vi "CV.vi"(2 "Run uninterrupted?":bool, 3 "Device Category IN:":string(combo)="ATLAS18SS" caption="Device Category:", 4 "Batch No.:":string, 5 "Sensor Serial No.:":string, 6 "DB Serial No.:":string) -> (0 "Done!":bool)   [LabVIEW 2019]
doc: "Performs CV measurements according to ATLAS ITk Quality Control Specifications."
uses:
  general_VIs/globals/QC_MeasurementSetup.vi
  general_VIs/globals/QC_RunInformation.vi
  InstrControl/InstrumentSetup.vi
  InstrControl/Switching/Switching.lvclass
  InstrControl/SupplyControl/SupplyControl.lvclass
  InstrControl/LCRControl/LCRControl.lvclass
  InstrControl/ArduinoControl/ArduinoControl.lvclass
  <vilib>/Analysis/NI_AALBase.lvlib
  InstrControl/InstrControl.lvclass
panel:
  out "Measurement Configuration Tab":enum32{"CV Setup", "CV Scan"}(tab)
  in  "V_depletion limit [V]":dbl=-300.0
  in  "step interval [s] IN":i32=5 caption="step interval [s]"
  in  "step [V] IN":dbl=10.0 caption="step [V]" format="%.1f"
  in  "Final volts [V] IN":dbl=-500.0 caption="Final volts [V]"
  in  "Initial volts [V] IN":dbl caption="Initial volts [V]"
  in  "Current Limit [µA]":dbl=1000.0 min=0.0001 format="%.3f"
  in  "Continue":bool
  in  "Quit":bool
  in  "Software current limit?":bool
  in  "Frequency [Hz] Setup":i32=500 caption="Frequency [Hz]" format="%#.3p"
  in  "Measurement Configurations":bool
  out "RH":dbl[](array[numeric]) caption="RH [%]" format="%#.2f"
  out "step interval [s]":u32=5
  out "step [V]":dbl=10.0 format="%.1f"
  out "Final volts [V]":dbl=-700.0 format="%.1f"
  out "Initial volts [V]":dbl format="%.1f"
  out "Frequency [Hz]":i32=1000 format="%#.3p"
  out "Temp.":dbl[](array[numeric]) caption="Temp. [°C]" format="%#.2f"
  out "Volts":dbl[](array[numeric]) caption="Volts [V]"
  out "Resistance":dbl[](array[numeric]) caption="Res [kOhm]"
  out "Capacitance":dbl[](array[numeric]) caption="Cap [pF]"
  out "Cgraph":cluster{"Initial volts":dbl, dbl, dbl[]}(graph)
  in  "Scales":T1(ring)
  in  "Cscale":enum16{"1/C^2 [1/nF^2]", "nF", "pF"}(ring)
  out "positive ramp?":bool
  out "DUT Description/Hardware Tab":enum32{"CV Setup", "CV Scan"}(tab)
  in  "Switching":string(combo)="Pickering Matrix"
  in  "LCR Meter":string(combo)="WayneKerr 6440B"
  in  "User:":string(combo)="Christoph"
  in  "CV Supply":string(combo)="Keithley 2410"
  in  "Hardware Configurations":bool
  in  "Temperature":enum16{"Read Arduino", "Enter manually"}(ring)
  in  "Manufacturer:":string(combo)="Hamamatsu"
  in  "abort":bool
  out "Device Category:":string
  out "DB Serial No.:":string
  out "Current Volts:":dbl format="%.2f"
  in  "quit (no save)":bool
  in  "Quit & Save":bool
  out "Bias On/Off:":bool
  out "STATUS 1":string
  out "Initiated:":string
  out "Sensor No.:":string
  out "No of steps":u32
  out "Current reading No.":u32
  out "Last reading at:":string
  # "Strip Sensor QC: CV"
  # "University of\nCambridge"
  # "Vertical Scale:"
  # "Measurement Configuration"
  # "CV Scan parameters:"
  # "Last 5 readings:"
  # "n-4"
  # "n-3"
  # "n-2"
  # "n-1"
  # "n"
  # "DUT Description"
  # "Hardware"
  # "DUT & Test Description:"
  # "Current status:"
  # "Rdg No:"
  # "out of"
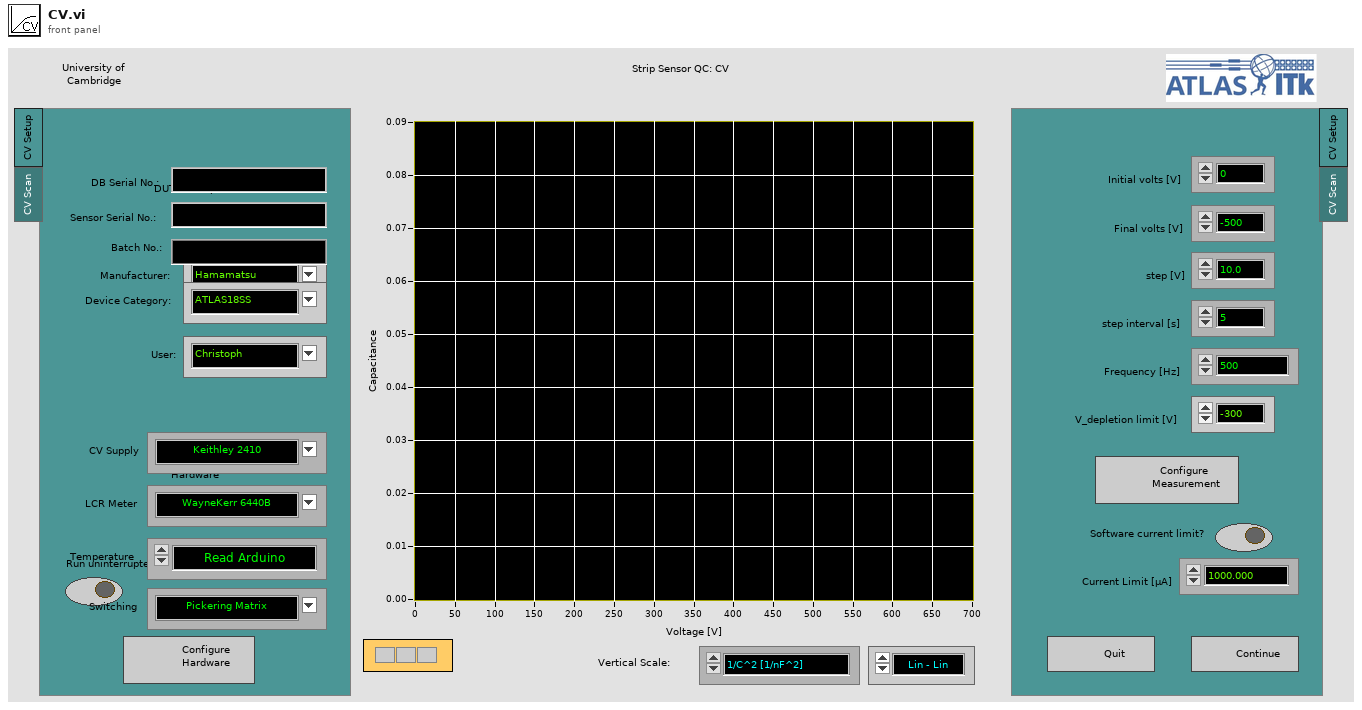
[diagram p1: front panel]
types:
  T1 = enum16{"Lin - Lin", "Log - Lin", "Lin - Log", "Log - log"}
  T2 = enum16{"Supply", "LCR", "Multimeter", "Switching"}
  T3 = enum16{"Reset", "Read Array", "Read Element", "Write Element", "Write Array", "Add Element", "Add Array"}
  T4 = enum16{"Reset", "Ground", "Striptest Bias", "Striptest SMU", "Striptest LCR", "IV", "CV", "Interstrip Cap", "Interstrip Res"}
  T5 = enum32{"IV", "CV", "Stability", "Striptest", "Cis", "Ris", "PTP"}
  T6 = cluster{"Supply":refnum<class "SupplyControl.lvclass">, "LCR":refnum<class "LCRControl.lvclass">, "Initial Voltage [V]":dbl, "Final Voltage [V]":dbl, "Step Size [V]":dbl, "Step Interval [s]":i32, "Number Of Steps":u32, "AC frequency [Hz]":i32, "RC Configuration":u16, "AC amplitude [V]":dbl, "Ramp down steps [V]":dbl, "Ramp down Interval [s]":i32, "Set Current Limit?":bool, "Current Limit [µA]":dbl, "Temperature Readout":enum16{"Read Arduino", "Enter manually"}, "Arduino":refnum<class "ArduinoControl.lvclass">, "Supply Name":string, "LCR Name":string, "V_depletion Limit [V]":dbl, "Switching":refnum<class "Switching.lvclass">, "Matrix used?":bool, "Matrix X Channels":cluster{"Bias Supply / SMU LO":i32, "Bias Supply / SMU HI":i32, "CV Box LO":i32, "CV Box HI":i32, "CV Box LO IN":i32, "CV Box HI IN":i32, "Volt meter LO":i32, "Volt meter HI":i32, "Mux1 C1":i32, "Mux1 C2":i32, "Mux2 C1":i32, "Mux2 C2":i32}}
  T7 = cluster{"Sensor Serial No.:":string, "Wafer Serial No.:":string, "Batch:":string, "Manufacturer:":string, "Device Category:":string, "Database Serial No.:":string, "Date Initiated:":string, "Time Initiated:":string, "Test":string, "Instruments used:":string, "Probeplan used:":string, "End of Run comment:":string, "User:":string}
  T8 = cluster{"Institute":string, "Manufacturers":string[], "Devices":string[], "Serialnumbers Lookup DB":string, "Data directory":string, "Backup & screenshot directory":string, "List of known users":string[], "Measurement switch not used":bool, "Measurement Switch":string, "DUT Switch":string}
  T9 = cluster{"Current Limit":sgl, "KE2410":refnum<class "KE2410.lvclass">}
  T10 = cluster{"VISA address":refnum<visa-resource-name>, "T sensor":enum16{"SHT", "DS"}, "Arduino":refnum<class "ArduinoControl.lvclass">}
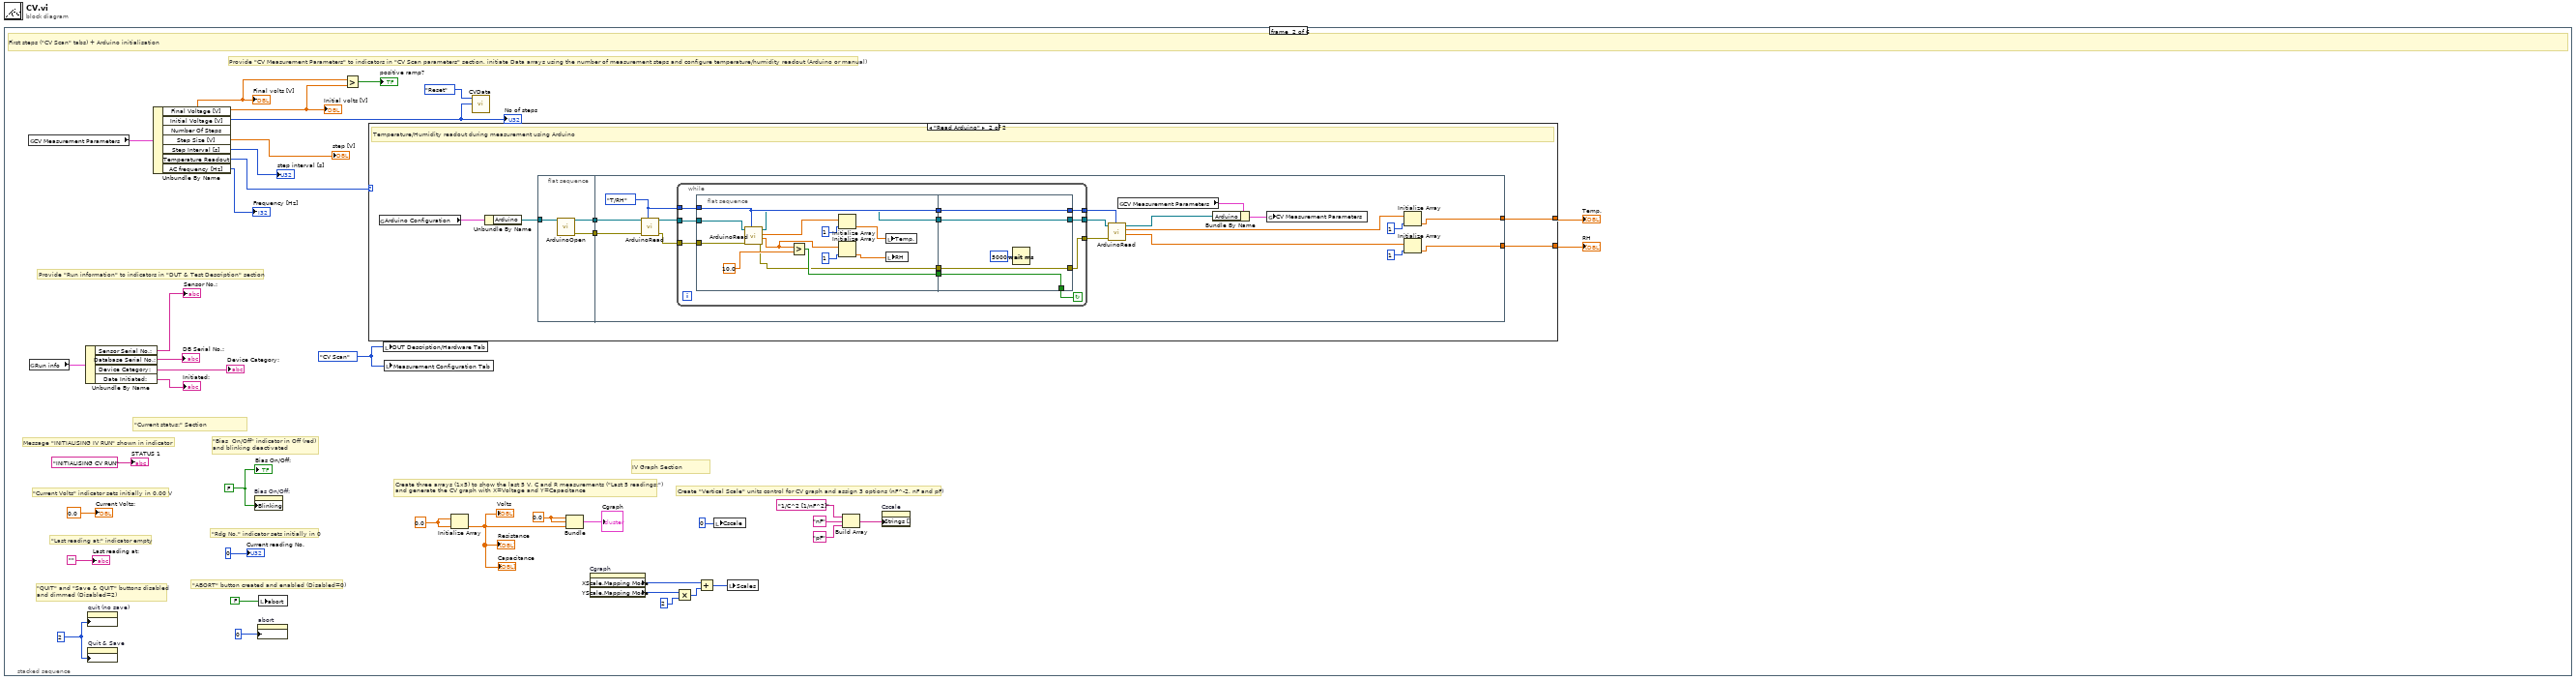
[diagram p0: block diagram]
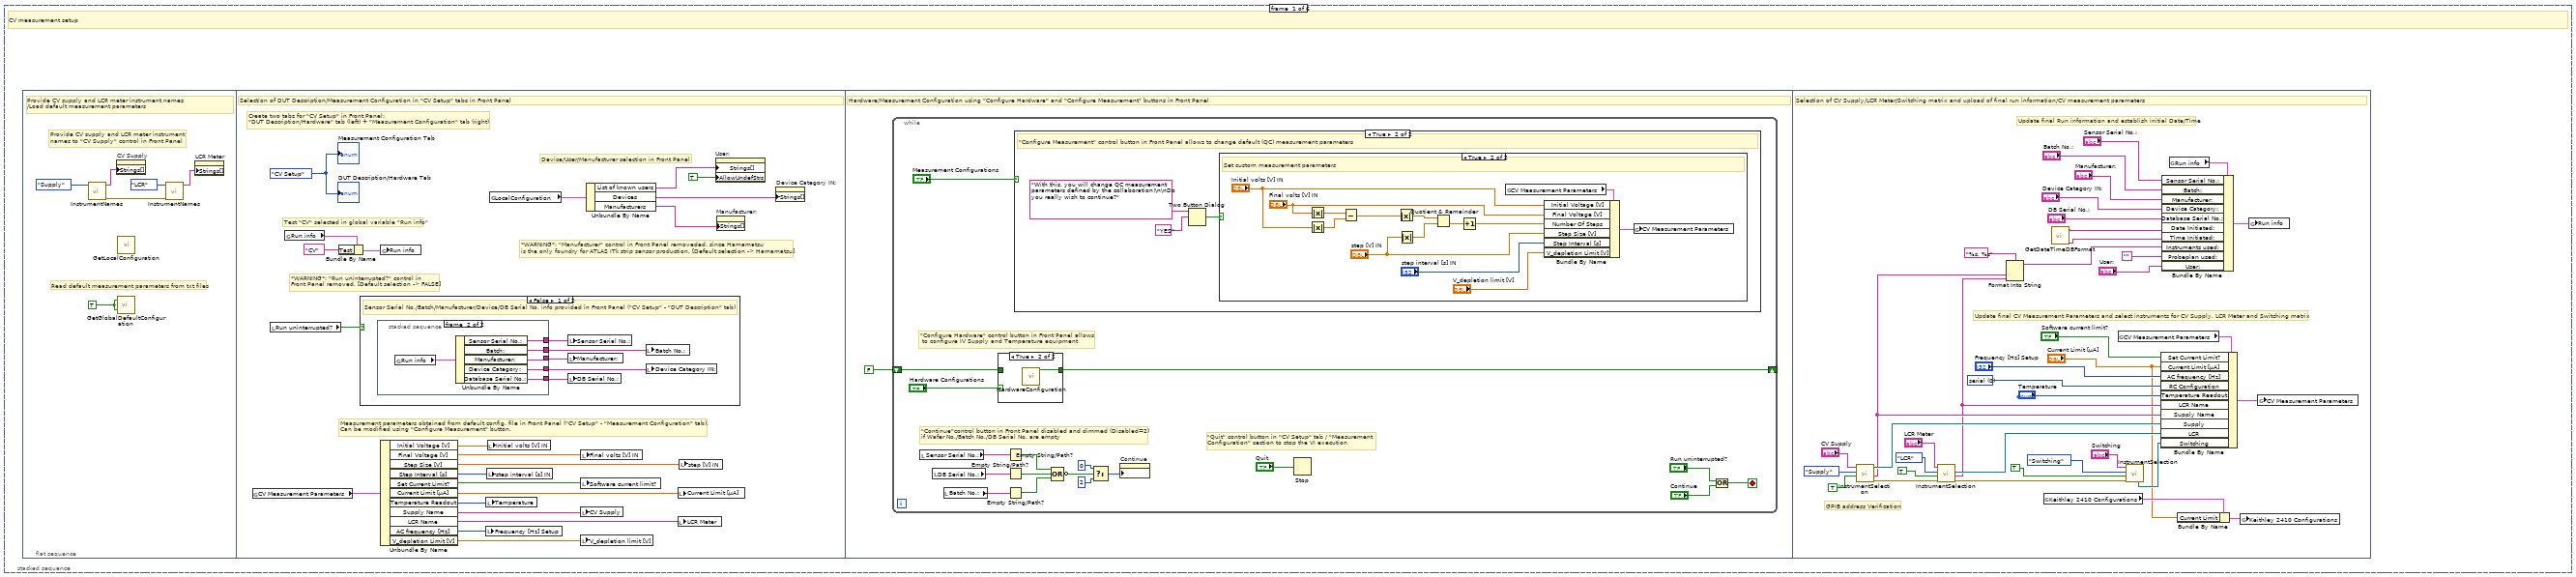
[diagram p2: hidden frame]
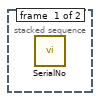
[diagram p3: hidden frame]
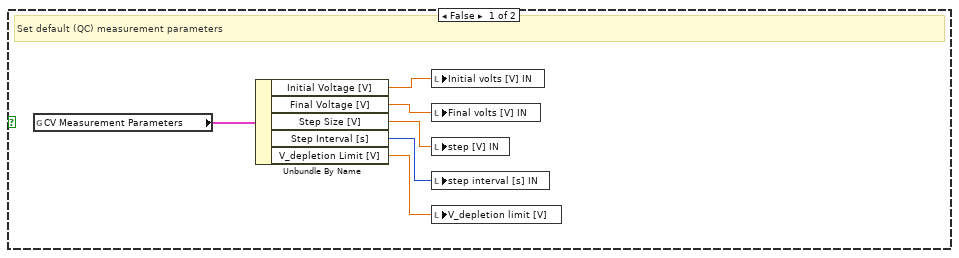
[diagram p7: hidden frame]
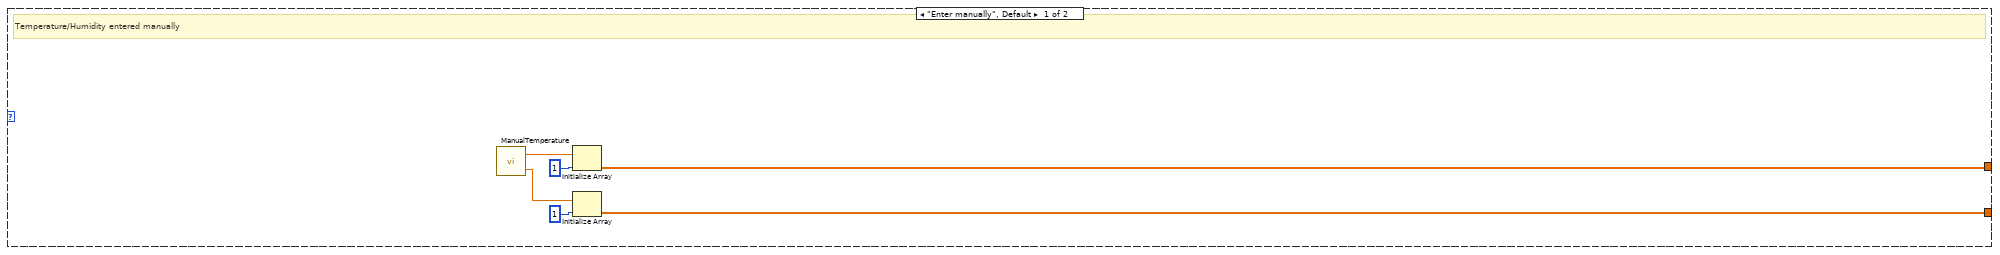
[diagram p8: hidden frame]
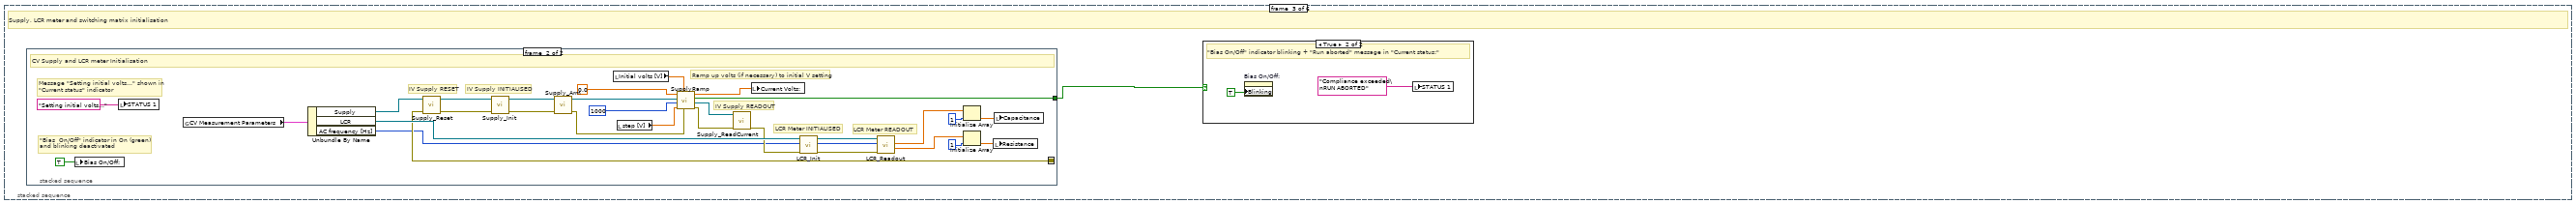
[diagram p9: hidden frame]
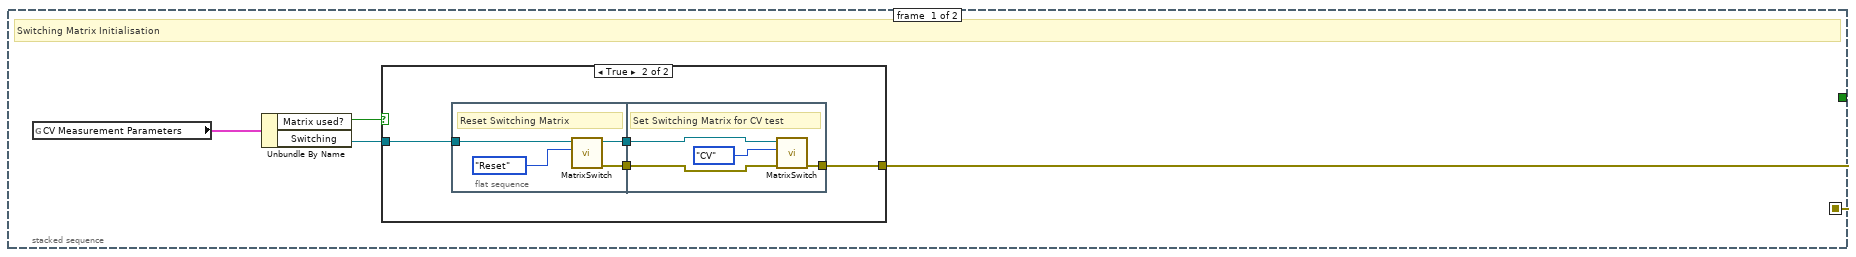
[diagram p10: hidden frame]
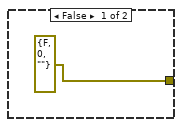
[diagram p11: hidden frame]
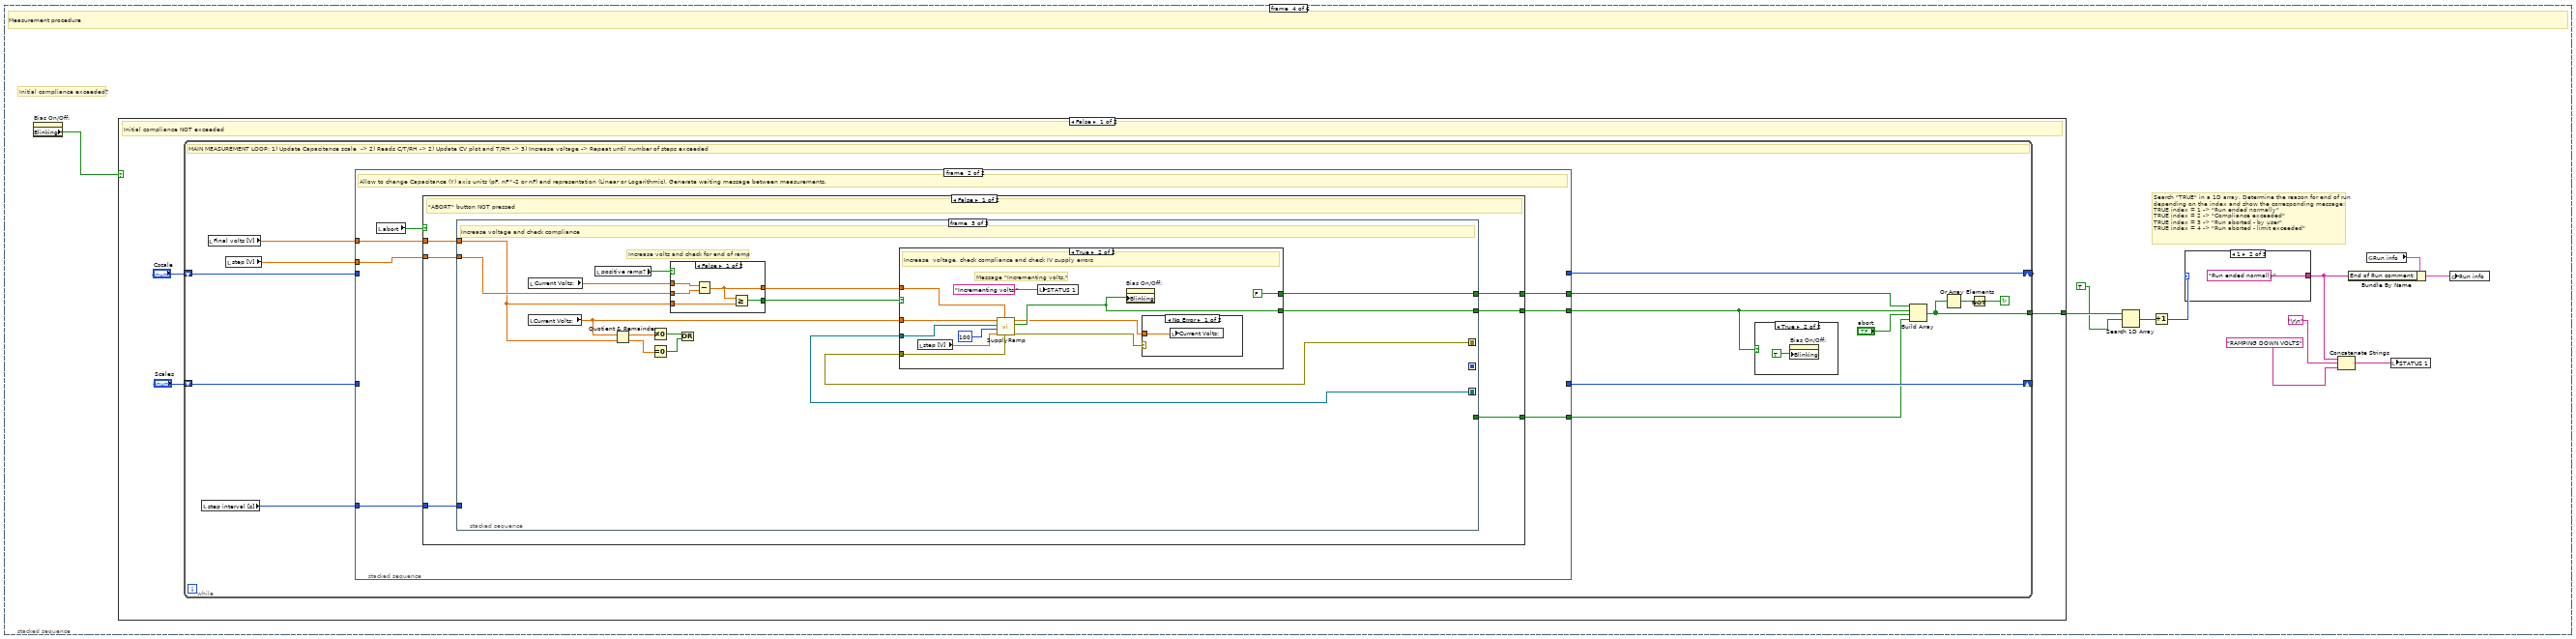
[diagram p13: hidden frame]
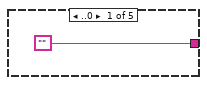
[diagram p14: hidden frame]
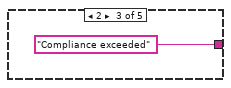
[diagram p15: hidden frame]
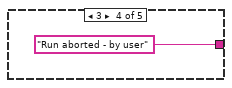
[diagram p16: hidden frame]
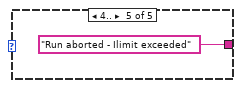
[diagram p17: hidden frame]
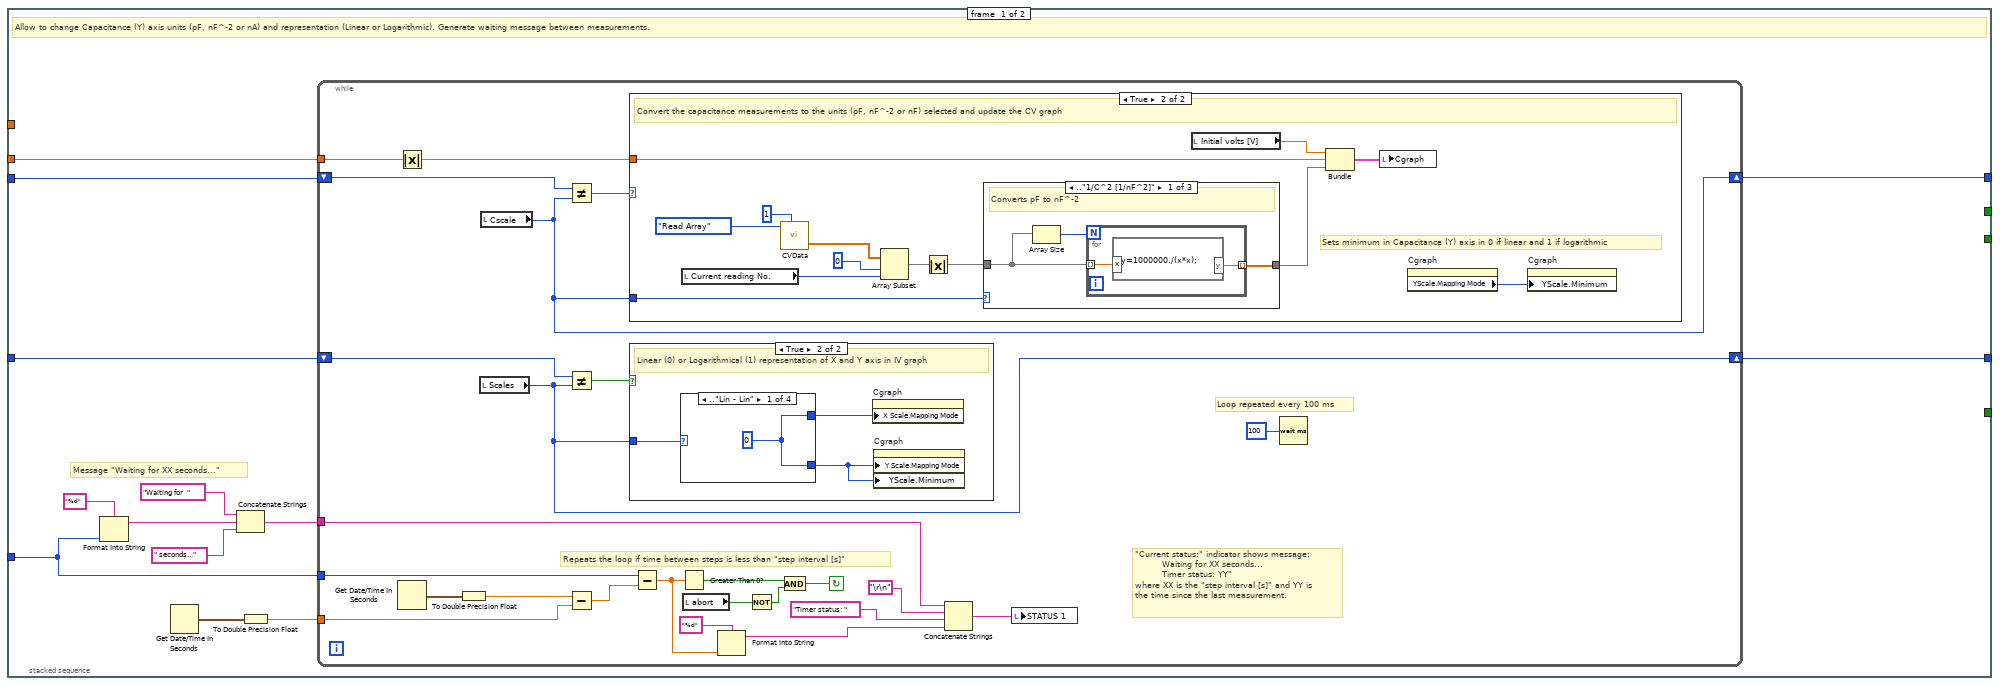
[diagram p18: hidden frame]
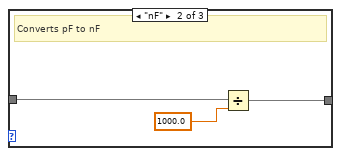
[diagram p20: hidden frame]
diagram:
  n1 = stacked-sequence {
    frame #0 {
      # "CV measurement setup"
      n2 = flat-sequence {
        frame #0 {
          w6 = TRUE
          # "Read default measurement parameters from txt files"
          # "Provide CV supply and LCR meter instrument \nnames to \"CV Supply\" control in Front Panel"
          # "Provide CV supply and LCR meter instrument names\n/Load default measurement parameters"
          n3 = call "InstrumentNames.vi"("Instrument type"=T2."Supply") -> ("error out"=w1:errorcluster, "Instrument names"=w3:string[])  [unwired: 9 in]
          n4 = property on="CV Supply" class="CmbBox"("Strings[]"=w3) -> ()  [unwired: 2 in, 2 out]
          n5 = call "GetGlobalDefaultConfiguration.vi"("DO NOT override instruments"=w6, "Read defaults?"=w6) -> ()  [unwired: 1 in, 1 out]
          n6 = call "GetLocalConfiguration.vi"() -> ()  [unwired: 3 in, 1 out]
          n7 = call "InstrumentNames.vi"("error in (no error)"=w1, "Instrument type"=T2."LCR") -> ("Instrument names"=w2:string[])  [unwired: 8 in, 1 out]
          n8 = property on="LCR Meter" class="CmbBox"("Strings[]"=w2) -> ()  [unwired: 2 in, 2 out]
        }
        frame #1 {
          w14 = enum32{"CV Setup", "CV Scan"}."CV Setup" ("Tab Control")
          # "Measurement parameters obtained from default config. file in Front Panel (\"CV Setup\" - \"Measurement Configuration\" tab).\nCan be modified using \"Configure Measurement\" button."
          # "*WARNING*: \"Run uninterrupted?\" control in \nFront Panel removed. [Default selection -> FALSE]"
          # "*WARNING*: \"Manufacturer\" control in Front Panel removeded, since Hamamatsu \nis the only foundry for ATLAS ITk strip sensor production. [Default selection -> Hamamatsu]"
          # "Test \"CV\" selected in global variable \"Run info\""
          # "Device/User/Manufacturer selection in Front Panel"
          # "Create two tabs for \"CV Setup\" in Front Panel:\n\"DUT Description/Hardware\" tab (left) + \"Measurement Configuration\" tab (right)"
          # "Selection of DUT Description/Measurement Configuration in \"CV Setup\" tabs in Front Panel"
          n9 = global read "QC_MeasurementSetup.vi" "CV Measurement Parameters"() -> (w26:T6)
          n10 = local read "Run uninterrupted?"() -> (w16:bool)
          n11 = global read "QC_RunInformation.vi" "Run info"() -> (w15:T7)
          n12 = Bundle By Name(cluster=w15, "Test"="CV") -> (w18:T7)
          n13 = case shown="False" w16 {
            frame False {
              # "Sensor Serial No./Batch/Manufacturer/Device/DB Serial No. info provided in Front Panel (\"CV Setup\" - \"DUT Description\" tab)"
              n14 = stacked-sequence {
                tunnel: [_ w39] -> w32
                tunnel: [_ w38] -> w31
                tunnel: [_ w37] -> w30
                tunnel: [_ w36] -> w33
                tunnel: [_ w34] -> w29
                frame #0 {
                  n15 = call "SerialNo.vi"() -> ()  [unwired: 5 in, 1 out]
                }
                frame #1 {
                  n16 = global read "QC_RunInformation.vi" "Run info"() -> (w35:T7)
                  n17 = Unbundle By Name(w35) -> ("Sensor Serial No.:"=w39:string, "Batch:"=w38:string, "Manufacturer:"=w37:string, "Device Category:"=w36:string, "Database Serial No.:"=w34:string)
                }
              }
              n18 = local write "Sensor Serial No.:"(w32) -> ()
              n19 = local write "Manufacturer:"(w30) -> ()
              n20 = local write "DB Serial No.:"(w29) -> ()
              n21 = local write "Batch No.:"(w31) -> ()
              n22 = local write "Device Category IN:"(w33) -> ()
            }
            frame True {
            }
          }
          n23 = global write "QC_RunInformation.vi" "Run info"(w18) -> ()
          n24 = Unbundle By Name(w26) -> ("Initial Voltage [V]"=w10:dbl, "Final Voltage [V]"=w11:dbl, "Step Size [V]"=w12:dbl, "Step Interval [s]"=w13:i32, "Set Current Limit?"=w25:bool, "Current Limit [µA]"=w24:dbl, "Temperature Readout"=w28:enum16{"Read Arduino", "Enter manually"}, "Supply Name"=w27:string, "LCR Name"=w20:string, "AC frequency [Hz]"=w19:i32, "V_depletion Limit [V]"=w9:dbl)
          n25 = local write "Frequency [Hz] Setup"(w19) -> ()
          n26 = local write "Temperature"(w28) -> ()
          n27 = local write "step interval [s] IN"(w13) -> ()
          n28 = local write "Initial volts [V] IN"(w10) -> ()
          n29 = global read "QC_RunInformation.vi" "LocalConfiguration"() -> (w23:T8)
          n30 = local write "CV Supply"(w27) -> ()
          n31 = local write "V_depletion limit [V]"(w9) -> ()
          n32 = local write "Final volts [V] IN"(w11) -> ()
          n33 = local write "Software current limit?"(w25) -> ()
          n34 = Unbundle By Name(w23) -> ("List of known users"=w22:string[], "Devices"=w7:string[], "Manufacturers"=w8:string[])
          n35 = local write "Current Limit [µA]"(w24) -> ()
          n36 = local write "LCR Meter"(w20) -> ()
          n37 = local write "step [V] IN"(w12) -> ()
          n38 = property on="User:" class="CmbBox"("Strings[]"=w22, "AllowUndefStrs"=TRUE) -> ()  [unwired: 2 in, 2 out]
          n39 = property on="Manufacturer:" class="CmbBox"("Strings[]"=w8) -> ()  [unwired: 2 in, 2 out]
          n40 = property on="Device Category IN:" class="CmbBox"("Strings[]"=w7) -> ()  [unwired: 2 in, 2 out]
          "DUT Description/Hardware Tab" <- w14
          "Measurement Configuration Tab" <- w14
        }
        frame #2 {
          # "Hardware/Measurement Configuration using \"Configure Hardware\" and \"Configure Measurement\" buttons in Front Panel"
          n41 = while {
            shift-right: [w41] -> _
            shift-left: FALSE -> [w43]
            stop <- w45 stop-if-true
            # "\"Configure Hardware\" control button in Front Panel allows\n to configure IV Supply and Temperature equipment"
            # "\"Continue\"control button in Front Panel disabled and dimmed (Disabled=2) \nif Wafer No./Batch No./DB Serial No. are empty"
            # "\"Quit\" control button in \"CV Setup\" tab / \"Measurement \nConfiguration\" section to stop the VI execution"
            n42 = local read "Sensor Serial No.:"() -> (w57:string)
            n43 = local read "DB Serial No.:"() -> (w56:string)
            n44 = local read "Batch No.:"() -> (w49:string)
            n45 = case shown="True" "Hardware Configurations" {
              tunnel: [w59 w60] -> w41
              tunnel: w43 -> [w59 _]
              frame False {
              }
              frame True {
                n46 = call "HardwareConfiguration.vi"() -> ("configured?"=w60:bool)  [unwired: 11 in]
              }
            }
            n47 = Empty String/Path?(string/path=w57) -> (empty?=w54:bool)
            n48 = Empty String/Path?(string/path=w56) -> (empty?=w55:bool)
            n49 = Empty String/Path?(string/path=w49) -> (empty?=w48:bool)
            n50 = case shown="True" "Measurement Configurations" {
              frame False {
              }
              frame True {
                # "\"Configure Measurement\" control button in Front Panel allows to change default (QC) measurement parameters"
                n51 = Two Button Dialog(message="With this, you will change QC measurement parameters defined by the collaboration!\n\nDo you really wish to continue?", 2:"YES") -> (T button?=w61:bool)  [unwired: 1 in]
                n52 = case shown="True" w61 {
                  frame False {
                    # "Set default (QC) measurement parameters"
                    n53 = global read "QC_MeasurementSetup.vi" "CV Measurement Parameters"() -> (w69:T6)
                    n54 = Unbundle By Name(w69) -> ("Initial Voltage [V]"=w66:dbl, "Final Voltage [V]"=w65:dbl, "Step Size [V]"=w67:dbl, "Step Interval [s]"=w68:i32, "V_depletion Limit [V]"=w64:dbl)
                    n55 = local write "Initial volts [V] IN"(w66) -> ()
                    n56 = local write "Final volts [V] IN"(w65) -> ()
                    n57 = local write "step [V] IN"(w67) -> ()
                    n58 = local write "step interval [s] IN"(w68) -> ()
                    n59 = local write "V_depletion limit [V]"(w64) -> ()
                  }
                  frame True {
                    # "Set custom measurement parameters"
                    n60 = Absolute Value(x="Final volts [V] IN") -> (abs(x)=w76:dbl)
                    n61 = Absolute Value(x="Initial volts [V] IN") -> (abs(x)=w77:dbl)
                    n62 = Subtract(x=w76, y=w77) -> (x-y=w80:dbl)
                    n63 = Absolute Value(x=w80) -> (abs(x)=w78:dbl)
                    n64 = Absolute Value(x="step [V] IN") -> (abs(x)=w79:dbl)
                    n65 = Quotient & Remainder(x=w78, y=w79) -> (floor(x/y)=w75:dbl)  [unwired: 1 out]
                    n66 = Increment(x=w75) -> (x+1=w71:dbl)
                    n67 = global read "QC_MeasurementSetup.vi" "CV Measurement Parameters"() -> (w83:T6)
                    n68 = Bundle By Name(cluster=w83, "Initial Voltage [V]"="Initial volts [V] IN", "Final Voltage [V]"="Final volts [V] IN", "Number Of Steps"=w71, "Step Size [V]"="step [V] IN", "Step Interval [s]"="step interval [s] IN", "V_depletion Limit [V]"="V_depletion limit [V]") -> (w82:T6)
                    n69 = global write "QC_MeasurementSetup.vi" "CV Measurement Parameters"(w82) -> ()
                  }
                }
              }
            }
            n70 = Compound Arithmetic op=OR(w54, w55, w48) -> (invert w53:bool)
            n71 = Select(t=0, s=w53, f=2) -> (s? t:f=w50:i32)
            n72 = property on="Continue" class="Bool"("DisabledEnum"=w50) -> ()  [unwired: 2 in, 2 out]
            n73 = Stop(stop? (T)="Quit") -> ()
            n74 = Or(x="Run uninterrupted?", y="Continue") -> (x .or. y?=w45:bool)
          }
        }
        frame #3 {
          w112 = u16 0 items=["serial", "parallel"] ("RC Configuration")
          # "Update final Run information and establish initial Date/Time"
          # "Update final CV Measurement Parameters and select instruments for CV Supply, LCR Meter and Switching matrix"
          # "GPIB address Verification"
          # "Selection of CV Supply/LCR Meter/Switching matrix and upload of final run information/CV measurement parameters"
          n75 = call "InstrumentSelection.vi"("Verify GPIB address"=TRUE, "Instrument type"=T2."Supply", "Instrument name IN"="CV Supply") -> ("error out"=w106:errorcluster, "Instrument name OUT"=w90:string, "Supply"=w105:refnum<class "SupplyControl.lvclass">)  [unwired: 3 in, 3 out]
          n76 = call "InstrumentSelection.vi"("error in (no error)"=w106, "Verify GPIB address"=TRUE, "Instrument type"=T2."LCR", "Instrument name IN"="LCR Meter") -> ("error out"=w102:errorcluster, "Instrument name OUT"=w89:string, "LCR"=w104:refnum<class "LCRControl.lvclass">)  [unwired: 2 in, 3 out]
          n77 = Format Into String(format string="%s, %s", w90, w89) -> (resulting string=w109:string)  [unwired: 2 in, 1 out]
          n78 = global read "InstrumentSetup.vi" "Keithley 2410 Configurations"() -> (w85:T9)
          n79 = call "GetDateTimeDBFormat.vi"() -> ("Time in 24h format, e.g. 13:40:54"=w87:string, "Abbreviated Date, e.g. 13 Nov 2020"=w88:string)  [unwired: 10 in]
          n80 = global read "QC_MeasurementSetup.vi" "CV Measurement Parameters"() -> (w120:T6)
          n81 = call "InstrumentSelection.vi"("error in (no error)"=w102, "Verify GPIB address"=TRUE, "Instrument type"=T2."Switching", "Instrument name IN"="Switching") -> ("Switching"=w101:refnum<class "Switching.lvclass">)  [unwired: 2 in, 5 out]
          n82 = Bundle By Name(cluster=w120, "Set Current Limit?"="Software current limit?", "Current Limit [µA]"="Current Limit [µA]", "AC frequency [Hz]"="Frequency [Hz] Setup", "RC Configuration"=w112, "Temperature Readout"="Temperature", "LCR Name"=w89, "Supply Name"=w90, "Supply"=w105, "LCR"=w104, "Switching"=w101) -> (w121:T6)
          n83 = global read "QC_RunInformation.vi" "Run info"() -> (w118:T7)
          n84 = Bundle By Name(cluster=w118, "Sensor Serial No.:"="Sensor Serial No.:", "Batch:"="Batch No.:", "Manufacturer:"="Manufacturer:", "Device Category:"="Device Category IN:", "Database Serial No.:"="DB Serial No.:", "Date Initiated:"=w88, "Time Initiated:"=w87, "Instruments used:"=w109, "Probeplan used:"="", "User:"="User:") -> (w117:T7)
          n85 = Bundle By Name(cluster=w85, "Current Limit"="Current Limit [µA]") -> (w86:T9)
          n86 = global write "InstrumentSetup.vi" "Keithley 2410 Configurations"(w86) -> ()
          n87 = global write "QC_RunInformation.vi" "Run info"(w117) -> ()
          n88 = global write "QC_MeasurementSetup.vi" "CV Measurement Parameters"(w121) -> ()
        }
      }
    }
    frame #1 {
      w124 = 0.0
      w127 = enum32{"CV Setup", "CV Scan"}."CV Scan" ("Tab Control")
      w143 = 2
      w150 = 0.0
      w142 = FALSE ("Visible")
      # "Provide \"CV Measurement Parameters\" to indicators in \"CV Scan parameters\" section, initiate Data arrays using the number of measurement steps and configure temperature/humidity readout (Arduino or manual)"
      # "IV Graph Section"
      # "\"Current status:\" Section"
      # "Message \"INITIALISING IV RUN\" shown in indicator"
      # "Create \"Vertical Scale\" units control for CV graph and assign 3 options (nF^-2, nF and pF)"
      # "Create three arrays (1x5) to show the last 5 V, C and R measurements (\"Last 5 readings:\") \nand generate the CV graph with X=Voltage and Y=Capacitance"
      # "Provide \"Run information\" to indicators in \"DUT & Test Description\" section"
      # "\"Bias  On/Off\" indicator in Off (red)\nand blinking deactivated"
      # "\"Rdg No.\" indicator sets initially in 0"
      # "\"Current Volts\" indicator sets initially in 0.00 V"
      # "\"ABORT\" button created and enabled (Disabled=0)"
      # "\"Last reading at:\" indicator empty"
      # "\"QUIT\" and \"Save & QUIT\" buttons disabled\nand dimmed (Disabled=2)"
      # "First steps (\"CV Scan\" tabs) + Arduino initialisation"
      n89 = global read "QC_MeasurementSetup.vi" "CV Measurement Parameters"() -> (w133:T6)
      n90 = global read "QC_RunInformation.vi" "Run info"() -> (w160:T7)
      n91 = Unbundle By Name(w160) -> ("Sensor Serial No.:"=→"Sensor No.:":string, "Database Serial No.:"=→"DB Serial No.:":string, "Device Category:"=→"Device Category:":string, "Date Initiated:"=→"Initiated:":string)
      n92 = property on="quit (no save)" class="Bool"("DisabledEnum"=w143) -> ()  [unwired: 2 in, 2 out]
      n93 = property on="Quit & Save" class="Bool"("DisabledEnum"=w143) -> ()  [unwired: 2 in, 2 out]
      n94 = Unbundle By Name(w133) -> ("Final Voltage [V]"=w122:dbl, "Initial Voltage [V]"=w123:dbl, "Number Of Steps"=w151:u32, "Step Size [V]"=→"step [V]":dbl, "Step Interval [s]"=→"step interval [s]":i32, "Temperature Readout"=w144:enum16{"Read Arduino", "Enter manually"}, "AC frequency [Hz]"=→"Frequency [Hz]":i32)
      "No of steps" <- w151
      "Initial volts [V]" <- w123
      "Final volts [V]" <- w122
      n95 = property on="Bias On/Off:" class="Bool (strict)"("Blinking"=w142) -> ()  [unwired: 2 in, 2 out]
      n96 = property on="abort" class="Bool (strict)"("DisabledEnum"=0) -> ()  [unwired: 2 in, 2 out]
      n97 = local write "abort"(FALSE) -> ()
      n98 = Greater?(x=w122, y=w123) -> (0:→"positive ramp?":bool)
      n99 = case shown="\"Read Arduino\"" w144 {
        tunnel: [w166 w173] -> w147
        tunnel: [w163 w172] -> w134
        frame "Enter manually", Default {
          # "Temperature/Humidity entered manually"
          n100 = call "ManualTemperature.vi"() -> ("Humidity [%] out"=w162:dbl, "Temperature [°C] out"=w167:dbl)
          n101 = Initialize Array(w167, 1) -> (w166:dbl[])
          n102 = Initialize Array(w162, 1) -> (w163:dbl[])
        }
        frame "Read Arduino" {
          # "Temperature/Humidity readout during measurement using Arduino"
          n103 = global read "InstrumentSetup.vi" "Arduino Configuration"() -> (w169:T10)
          n104 = Unbundle By Name(w169) -> ("Arduino"=w168:refnum<class "ArduinoControl.lvclass">)
          n105 = flat-sequence {
            tunnel: [w174] -> w171
            tunnel: [w176] -> w170
            tunnel: w168 -> [w175]
            tunnel: [w193] -> w173
            tunnel: [w190] -> w172
            tunnel: w171 -> [w183]
            tunnel: w170 -> [w184]
            frame #0 {
              n106 = call "ArduinoOpen.vi"("ArduinoControl in"=w175) -> ("error out"=w176:errorcluster, "ArduinoControl out"=w174:refnum<class "ArduinoControl.lvclass">)  [unwired: 9 in]
            }
            frame #1 {
              w180 = enum16{"T/RH", "Interlock", "Edgesense"}."T/RH" ("Arduino function")
              n107 = call "ArduinoRead.vi"("Arduino function"=w180, "error in (no error)"=w184, "ArduinoControl in"=w183) -> ("error out"=w182:errorcluster, "ArduinoControl out"=w181:refnum<class "ArduinoControl.lvclass">)  [unwired: 3 in, 4 out]
              n108 = while {
                tunnel: w181 -> [w204]
                tunnel: w182 -> [w203]
                tunnel: w180 -> [w202]
                tunnel: [w200] -> w179
                tunnel: [w196] -> w178
                tunnel: [w194] -> w177
                stop <- w199 continue-if-true
                n109 = flat-sequence {
                  tunnel: w204 -> [w212]
                  tunnel: w203 -> [w211]
                  tunnel: w202 -> [w210]
                  tunnel: [w210] -> w201
                  tunnel: [w209] -> w198
                  tunnel: [w208] -> w197
                  tunnel: [w207] -> w195
                  tunnel: [w222] -> w200
                  tunnel: w201 -> [w222]
                  tunnel: [w221] -> w199
                  tunnel: w198 -> [w221]
                  tunnel: [w219] -> w196
                  tunnel: w197 -> [w219]
                  tunnel: [w218] -> w194
                  tunnel: w195 -> [w218]
                  frame #0 {
                    n110 = call "ArduinoRead.vi"("Arduino function"=w210, "error in (no error)"=w211, "ArduinoControl in"=w212) -> ("error out"=w208:errorcluster, "rel. Humidity [%]"=w214:dbl, "Temperature [°C]"=w213:dbl, "ArduinoControl out"=w207:refnum<class "ArduinoControl.lvclass">)  [unwired: 3 in, 2 out]
                    n111 = Greater?(x=w214, y=10.0 ("Start Humidity")) -> (0:w209:bool)
                    n112 = Initialize Array(w213, 1) -> (w205:dbl[])
                    n113 = Initialize Array(w214, 1) -> (w206:dbl[])
                    n114 = local write "Temp."(w205) -> ()
                    n115 = local write "RH"(w206) -> ()
                  }
                  frame #1 {
                    n116 = Wait (ms)(milliseconds to wait=u32 5000) -> ()  [unwired: 1 out]
                  }
                }
              }
              n117 = call "ArduinoRead.vi"("Arduino function"=w179, "error in (no error)"=w178, "ArduinoControl in"=w177) -> ("rel. Humidity [%]"=w188:dbl, "Temperature [°C]"=w189:dbl, "ArduinoControl out"=w187:refnum<class "ArduinoControl.lvclass">)  [unwired: 3 in, 3 out]
              n118 = global read "QC_MeasurementSetup.vi" "CV Measurement Parameters"() -> (w186:T6)
              n119 = Bundle By Name(cluster=w186, "Arduino"=w187) -> (w185:T6)
              n120 = global write "QC_MeasurementSetup.vi" "CV Measurement Parameters"(w185) -> ()
              n121 = Initialize Array(w189, 1) -> (w193:dbl[])
              n122 = Initialize Array(w188, 1) -> (w190:dbl[])
            }
          }
        }
      }
      "Temp." <- w147
      "RH" <- w134
      n123 = local write "DUT Description/Hardware Tab"(w127) -> ()
      n124 = local write "Measurement Configuration Tab"(w127) -> ()
      n125 = Initialize Array(w150, w150) -> (w129:dbl[])
      "Volts" <- w129
      "Capacitance" <- w129
      "Resistance" <- w129
      n126 = call "CVData.vi"("Action"=T3."Reset", "Array Size / Index"=w151) -> ()  [unwired: 3 in, 2 out]
      n127 = Bundle(w124, w124, w129) -> (→"Cgraph":cluster{dbl, dbl, dbl[]})  [unwired: 1 in]
      n128 = property on="Cgraph" class="WFGraph (strict)"() -> ("XScale.Mapping Mode"=w137:u8, "YScale.Mapping Mode"=w136:u8)  [unwired: 2 in, 2 out]
      n129 = Multiply(x=w136, y=2) -> (x*y=w139:i32)
      n130 = Add(x=w137, y=w139) -> (x+y=w135:i32)
      n131 = local write "Cscale"(u16 0 ("Scale")) -> ()
      n132 = local write "Scales"(w135) -> ()
      n133 = Build Array("1/C^2 [1/nF^2]", "nF", "pF") -> (w157:string[])
      n134 = property on="Cscale" class="Enum (strict)"("Strings []"=w157) -> ()  [unwired: 2 in, 2 out]
      "STATUS 1" <- "INITIALISING CV RUN"
      "Bias On/Off:" <- w142
      "Last reading at:" <- ""
      "Current reading No." <- u32 0 ("Current reading No.")
      "Current Volts:" <- 0.0 ("Current Volts:")
    }
    frame #2 {
      # "Supply, LCR meter and switching matrix initialisation"
      n135 = stacked-sequence {
        seq-local: [w225 _] -> [_ w248]
        tunnel: [_ w252] -> w223
        frame #0 {
          # "Switching Matrix Initialisation"
          n136 = global read "QC_MeasurementSetup.vi" "CV Measurement Parameters"() -> (w224:T6)
          n137 = Unbundle By Name(w224) -> ("Matrix used?"=w227:bool, "Switching"=w226:refnum<class "Switching.lvclass">)
          n138 = case shown="True" w227 {
            tunnel: w226 -> [_ w229]
            tunnel: [errorcluster {"status"=FALSE, "code"=0, "source"=""} ("error constant") w230] -> w225
            frame False {
            }
            frame True {
              n139 = flat-sequence {
                tunnel: [w236] -> w232
                tunnel: [w235] -> w231
                tunnel: w229 -> [w234]
                tunnel: w232 -> [w240]
                tunnel: w231 -> [w239]
                tunnel: [w238] -> w230
                frame #0 {
                  # "Reset Switching Matrix"
                  n140 = call-dynamic "MatrixSwitch.vi"("Action"=T4."Reset", "Switching in"=w234) -> ("error out"=w236:errorcluster, "Switching out"=w235:refnum<class "Switching.lvclass">)  [unwired: 7 in, 1 out]
                }
                frame #1 {
                  # "Set Switching Matrix for CV test"
                  n141 = call-dynamic "MatrixSwitch.vi"("error in (no error)"=w240, "Action"=T4."CV", "Switching in"=w239) -> ("error out"=w238:errorcluster)  [unwired: 6 in, 2 out]
                }
              }
            }
          }
        }
        frame #1 {
          # "IV Supply READOUT"
          # "LCR Meter READOUT"
          # "LCR Meter INITIALISED"
          # "IV Supply INITIALISED"
          # "IV Supply RESET"
          # "Message \"Setting initial volts...\" shown in \n\"Current status\" indicator"
          # "\"Bias  On/Off\" indicator in On (green)\nand blinking deactivated"
          # "Ramp up volts (if necessary) to initial V setting"
          # "CV Supply and LCR meter Initialisation"
          n142 = local write "Bias On/Off:"(TRUE ("Compliance?")) -> ()
          n143 = local write "STATUS 1"("Setting initial volts..." ("STATUS 1")) -> ()
          n144 = global read "QC_MeasurementSetup.vi" "CV Measurement Parameters"() -> (w266:T6)
          n145 = Unbundle By Name(w266) -> ("Supply"=w263:refnum<class "SupplyControl.lvclass">, "LCR"=w262:refnum<class "LCRControl.lvclass">, "AC frequency [Hz]"=w241:i32)
          n146 = call-dynamic "Supply_Reset.vi"("error in (no error)"=w248, "SupplyControl in"=w263) -> ("error out"=w268:errorcluster, "SupplyControl out"=w270:refnum<class "SupplyControl.lvclass">)  [unwired: 8 in]
          n147 = call-dynamic "Supply_Init.vi"("error in (no error)"=w268, "SupplyControl in"=w270) -> ("error out"=w267:errorcluster, "SupplyControl out"=w269:refnum<class "SupplyControl.lvclass">)  [unwired: 8 in]
          n148 = call-dynamic "Supply_Arm.vi"("error in (no error)"=w267, "SupplyControl in"=w269) -> ("error out"=w250:errorcluster, "SupplyControl out"=w251:refnum<class "SupplyControl.lvclass">)  [unwired: 8 in]
          n149 = local read "Initial volts [V]"() -> (w255:dbl)
          n150 = local read "step [V]"() -> (w256:dbl)
          n151 = call "SupplyRamp.vi"("error in"=w250, "Requested Voltage"=w255, "Step Size"=w256, "Step Delay"=1000, "Supply IN"=w251, "Starting Voltage"=0.0) -> ("error out"=w253:errorcluster, "Supply OUT"=w254:refnum<class "SupplyControl.lvclass">, "Compliance exceeded"=w252:bool, "Current Voltage"=w259:dbl)  [unwired: 2 in]
          n152 = call-dynamic "Supply_ReadCurrent.vi"("error in (no error)"=w253, "SupplyControl in"=w254) -> ("error out"=w249:errorcluster)  [unwired: 7 in, 2 out]
          n153 = local write "Current Volts:"(w259) -> ()
          n154 = call-dynamic "LCR_Init.vi"("error in (no error)"=w249, "LCRControl in"=w262) -> ("error out"=w246:errorcluster, "LCRControl out"=w247:refnum<class "LCRControl.lvclass">)  [unwired: 8 in]
          n155 = call-dynamic "LCR_Readout.vi"("error in (no error)"=w246, "Frequency in Hz"=w241, "LCRControl in"=w247) -> ("Resistance in Ohm"=w243:dbl, "Capacitance in pF"=w245:dbl)  [unwired: 5 in, 2 out]
          n156 = Initialize Array(w245, 1) -> (w260:dbl[])
          n157 = Initialize Array(w243, 1) -> (w242:dbl[])
          n158 = local write "Resistance"(w242) -> ()
          n159 = local write "Capacitance"(w260) -> ()
        }
      }
      n160 = case shown="True" w223 {
        frame False {
        }
        frame True {
          # "\"Bias On/Off\" indicator blinking + \"Run aborted\" message in \"Current status:\""
          n161 = property on="Bias On/Off:" class="Bool (strict)"("Blinking"=TRUE) -> ()  [unwired: 2 in, 2 out]
          n162 = local write "STATUS 1"("Compliance exceeded\nRUN ABORTED") -> ()
        }
      }
    }
    frame #3 {
      # "Search \"TRUE\" in a 1D array. Determine the reason for end of run \ndepending on the index and show the corresponding message:\nTRUE index = 1 -> \"Run ended normally\"\nTRUE index = 2 -> \"Compliance exceeded\"\nTRUE index = 3 -> \"Run aborted - by user\"\nTRUE index = 4 -> \"Run aborted - limit exceeded\""
      # "Initial compliance exceeded?"
      # "Measurement procedure"
      n163 = property on="Bias On/Off:" class="Bool (strict)"() -> ("Blinking"=w283:bool)  [unwired: 2 in, 2 out]
      n164 = case shown="False" w283 {
        tunnel: [w291 w548] -> w282
        frame False {
          # "Initial compliance NOT exceeded"
          n165 = while {
            shift-left: "Cscale" -> [w301]
            shift-right: [w300] -> _
            shift-left: "Scales" -> [w302]
            shift-right: [w303] -> _
            tunnel: [w299] -> w291
            stop <- w304 continue-if-true
            # "MAIN MEASUREMENT LOOP: 1) Update Capacitance scale  -> 2) Reads C/T/RH -> 2) Update CV plot and T/RH -> 3) Increase voltage -> Repeat until number of steps exceeded"
            n166 = local read "step interval [s]"() -> (w296:u32)
            n167 = local read "Final volts [V]"() -> (w297:dbl)
            n168 = local read "step [V]"() -> (w298:dbl)
            n169 = stacked-sequence {
              tunnel: [w318 _] -> w303
              tunnel: w298 -> [w315 w381]
              tunnel: [_ w380] -> w293
              tunnel: w297 -> [_ w379]
              tunnel: w296 -> [w306 w378]
              tunnel: [_ w377] -> w295
              tunnel: w302 -> [w317 _]
              tunnel: w301 -> [w316 _]
              tunnel: [w314 _] -> w300
              tunnel: [_ w375] -> w294
              frame #0 {
                # "Message \"Waiting for XX seconds...\""
                # "Allow to change Capacitance (Y) axis units (pF, nF^-2 or nA) and representation (Linear or Logarithmic). Generate waiting message between measurements."
                n170 = Format Into String(format string="%d", w306) -> (resulting string=w311:string)  [unwired: 2 in, 1 out]
                n171 = Get Date/Time In Seconds() -> (seconds since 1Jan1904=w308:timestamp)
                n172 = Concatenate Strings("Waiting for  ", w311, " seconds...") -> (w307:string)
                n173 = To Double Precision Float(number=w308) -> (double precision float=w309:dbl)
                n174 = while {
                  tunnel: w315 -> [w327]
                  shift-left: w316 -> [w331]
                  shift-right: [w324] -> w314
                  shift-left: w317 -> [w332]
                  shift-right: [w333] -> w318
                  tunnel: w307 -> [w325]
                  tunnel: w306 -> [w337]
                  tunnel: w309 -> [w338]
                  stop <- w339 continue-if-true
                  # "Loop repeated every 100 ms"
                  # "\"Current status:\" indicator shows message:\n         Waiting for XX seconds...\n         Timer status: YY\"\nwhere XX is the \"step interval [s]\" and YY is\nthe time since the last measurement."
                  # "Repeats the loop if time between steps is less than \"step interval [s]\""
                  n175 = Absolute Value(x=w327) -> (abs(x)=w326:dbl)
                  n176 = Get Date/Time In Seconds() -> (seconds since 1Jan1904=w323:timestamp)
                  n177 = To Double Precision Float(number=w323) -> (double precision float=w343:dbl)
                  n178 = local read "Scales"() -> (w333:T1)
                  n179 = local read "Cscale"() -> (w324:enum16{"1/C^2 [1/nF^2]", "nF", "pF"})
                  n180 = Not Equal?(x=w331, y=w324) -> (x != y?=w322:bool)
                  n181 = Not Equal?(x=w332, y=w333) -> (x != y?=w334:bool)
                  n182 = Subtract(x=w343, y=w338) -> (x-y=w320:dbl)
                  n183 = case shown="True" w322 {
                    tunnel: w326 -> [_ w355]
                    tunnel: w324 -> [_ w348]
                    frame False {
                    }
                    frame True {
                      # "Sets minimum in Capacitance (Y) axis in 0 if linear and 1 if logarithmic"
                      # "Convert the capacitance measurements to the units (pF, nF^-2 or nF) selected and update the CV graph"
                      n184 = local read "Current reading No."() -> (w353:u32)
                      n185 = call "CVData.vi"("Action"=T3."Read Array", "Array No."=u32 1 ("Action")) -> ("Array OUT"=w344:dbl[])  [unwired: 3 in, 1 out]
                      n186 = Array Subset(array=w344, index=0, length=w353) -> (w351:dbl[])
                      n187 = Absolute Value(x=w351) -> (abs(x)=w349:dbl[])
                      n188 = case shown="..\"1/C^2 [1/nF^2]\"" w348 {
                        tunnel: [w359 w362 w365] -> w347
                        tunnel: w349 -> [w357 w364 w365]
                        frame .."1/C^2 [1/nF^2]" {
                          # "Converts pF to nF^-2"
                          n189 = Array Size(array=w357) -> (size(s)=w358:i32)
                          n190 = for {
                            N: w358 -> [_]
                            tunnel: w357 -> [w361] mode=indexing
                            tunnel: [w360] -> w359 mode=indexing
                            n191 = formula code="y=1000000./(x*x);"("x"=w361) -> ("y"=w360:dbl)
                          }
                        }
                        frame "nF" {
                          # "Converts pF to nF"
                          n192 = Divide(x=w364, y=1000.0) -> (x/y=w362:dbl[])
                        }
                        frame "pF".. {
                        }
                      }
                      n193 = local read "Initial volts [V]"() -> (w354:dbl)
                      n194 = Bundle("Initial volts [V]"=w354, w355, w347) -> (w352:cluster{"Initial volts [V]":dbl, dbl, dbl[]})  [unwired: 1 in]
                      n195 = local write "Cgraph"(w352) -> ()
                      n196 = property on="Cgraph" class="WFGraph (strict)"() -> ("YScale.Mapping Mode"=w350:u8)  [unwired: 2 in, 2 out]
                      n197 = property on="Cgraph" class="WFGraph (strict)"("YScale.Minimum"=w350) -> ()  [unwired: 2 in, 2 out]
                    }
                  }
                  n198 = case shown="True" w334 {
                    tunnel: w333 -> [_ w368]
                    frame False {
                    }
                    frame True {
                      # "Linear (0) or Logarithmical (1) representation of X and Y axis in IV graph"
                      n199 = case shown="..\"Lin - Lin\"" w368 {
                        tunnel: [w369 1 0 w374] -> w367
                        tunnel: [w369 0 1 w374] -> w366
                        frame .."Lin - Lin" {
                          w369 = 0
                        }
                        frame "Log - Lin" {
                        }
                        frame "Lin - Log" {
                        }
                        frame "Log - log".. {
                          w374 = 1
                        }
                      }
                      n200 = property on="Cgraph" class="WFGraph (strict)"("X Scale.Mapping Mode"=w367) -> ()  [unwired: 2 in, 2 out]
                      n201 = property on="Cgraph" class="WFGraph (strict)"("Y Scale.Mapping Mode"=w366, "YScale.Minimum"=w366) -> ()  [unwired: 2 in, 2 out]
                    }
                  }
                  n202 = Subtract(x=w337, y=w320) -> (x-y=w319:dbl)
                  n203 = Greater Than 0?(x=w319) -> (x > 0?=w321:bool)
                  n204 = local read "abort"() -> (w336:bool)
                  n205 = Format Into String(format string="%d", w319) -> (resulting string=w341:string)  [unwired: 2 in, 1 out]
                  n206 = Not(x=w336) -> (.not. x?=w342:bool)
                  n207 = And(x=w321, y=w342) -> (x .and. y?=w339:bool)
                  n208 = Concatenate Strings(w325, "\r\n", "Timer status: ", w341) -> (w335:string)
                  n209 = local write "STATUS 1"(w335) -> ()
                  n210 = Wait (ms)(milliseconds to wait=u32 100) -> ()  [unwired: 1 out]
                }
              }
              frame #1 {
                # "Allow to change Capacitance (Y) axis units (pF, nF^-2 or nF) and representation (Linear or Logarithmic). Generate waiting message between measurements."
                n211 = local read "abort"() -> (w376:bool)
                n212 = case shown="False" w376 {
                  tunnel: [w387 w545] -> w377
                  tunnel: w378 -> [w386 _]
                  tunnel: w379 -> [w385 _]
                  tunnel: [w383 w545] -> w380
                  tunnel: w381 -> [w384 _]
                  tunnel: [w382 w545] -> w375
                  frame False {
                    # "\"ABORT\" button NOT pressed"
                    n213 = stacked-sequence {
                      seq-local: [w422 _ _] -> [_ w446 _]
                      seq-local: [w421 _ _] -> [_ _ w514]
                      seq-local: [w413 _ _] -> [_ _ w515]
                      tunnel: w384 -> [_ w458 w520]
                      tunnel: w385 -> [_ _ w511]
                      tunnel: [_ _ w518] -> w387
                      tunnel: [_ _ w517] -> w383
                      tunnel: w386 -> [_ _ _]
                      tunnel: [w424 _ _] -> w382
                      frame #0 {
                        # "Increase in 1 the measurement number"
                        # "Write Relative Humidity [%] in 5th column"
                        # "Write Temperature [ºC] in 4th column"
                        # "Write Resistance [Ohm] in 3rd column"
                        # "Write Capacitance [pF] in 2nd column"
                        # "Convert to nA"
                        # "Write Voltage [V] in 1st column"
                        # "Show \"Reading current ...\" message \nin \"Current status:\" indicator"
                        # "Show date/time of last measurement \nin \"Last reading at:\" indicator"
                        # "READ and WRITE Voltage/Capacitance/Resistance/Temperature/Relative Humidity. Check Current compliance. Show date/time of last measurement and \"Reading current...\" message."
                        n214 = global read "QC_MeasurementSetup.vi" "CV Measurement Parameters"() -> (w403:T6)
                        n215 = Get Date/Time String(want seconds? (F)=TRUE) -> (time string=w423:string)  [unwired: 2 in, 1 out]
                        n216 = local write "Last reading at:"(w423) -> ()
                        n217 = local write "STATUS 1"("Reading LCR meter..." ("status")) -> ()
                        n218 = Unbundle By Name(w403) -> ("LCR"=w397:refnum<class "LCRControl.lvclass">, "AC frequency [Hz]"=w396:i32, "Supply"=w398:refnum<class "SupplyControl.lvclass">, "Set Current Limit?"=w399:bool, "Current Limit [µA]"=w400:dbl, "Arduino"=w401:refnum<class "ArduinoControl.lvclass">, "Temperature Readout"=w402:enum16{"Read Arduino", "Enter manually"})
                        n219 = call-dynamic "Supply_ReadCurrent.vi"("SupplyControl in"=w398) -> ("error out"=w414:errorcluster, "Current in nA"=w425:dbl, "SupplyControl out"=w421:refnum<class "SupplyControl.lvclass">)  [unwired: 8 in]
                        n220 = Multiply(x=w400, y=1000.0) -> (x*y=w419:dbl)
                        n221 = case shown="True" w399 {
                          tunnel: w425 -> [_ w442]
                          tunnel: w419 -> [_ w440]
                          tunnel: [FALSE w439] -> w424
                          frame False {
                          }
                          frame True {
                            # "Current > Compliance?"
                            n222 = Absolute Value(x=w442) -> (abs(x)=w441:dbl)
                            n223 = Greater?(x=w441, y=w440) -> (0:w439:bool)
                          }
                        }
                        n224 = case shown="\"Enter manually\", Default" w402 {
                          tunnel: [w431 w434] -> w407
                          tunnel: [w428 w437] -> w411
                          tunnel: w401 -> [_ w436]
                          frame "Enter manually", Default {
                            # "Read T/RH entered manually"
                            n225 = local read "Temp."() -> (w433:dbl[])
                            n226 = local read "RH"() -> (w429:dbl[])
                            n227 = Index Array(array=w433, index=0) -> (element=w431:dbl)
                            n228 = Index Array(array=w429, index=0) -> (element=w428:dbl)
                          }
                          frame "Read Arduino" {
                            # "Read  T/RH from Arduino"
                            n229 = call "ArduinoRead.vi"("Arduino function"=enum16{"T/RH", "Interlock", "Edgesense"}."T/RH", "ArduinoControl in"=w436) -> ("rel. Humidity [%]"=w437:dbl, "Temperature [°C]"=w434:dbl)  [unwired: 4 in, 4 out]
                          }
                        }
                        n230 = call-dynamic "LCR_Readout.vi"("error in (no error)"=w414, "Frequency in Hz"=w396, "LCRControl in"=w397) -> ("error out"=w413:errorcluster, "Resistance in Ohm"=w408:dbl, "Capacitance in pF"=w406:dbl)  [unwired: 5 in, 1 out]
                        n231 = local read "Current reading No."() -> (w389:u32)
                        n232 = local read "Current reading No."() -> (w392:u32)
                        n233 = local read "Current reading No."() -> (w391:u32)
                        n234 = local read "Current reading No."() -> (w394:u32)
                        n235 = local read "Current reading No."() -> (w405:u32)
                        n236 = local read "Current Volts:"() -> (w412:dbl)
                        n237 = call "CVData.vi"("Action"=T3."Write Element", "Array No."=u32 4, "Array Size / Index"=w389, "Data IN"=w411) -> ()  [unwired: 1 in, 2 out]
                        n238 = call "CVData.vi"("Action"=T3."Write Element", "Array No."=u32 3, "Array Size / Index"=w391, "Data IN"=w407) -> ()  [unwired: 1 in, 2 out]
                        n239 = call "CVData.vi"("Action"=T3."Write Element", "Array No."=u32 2, "Array Size / Index"=w392, "Data IN"=w408) -> ()  [unwired: 1 in, 2 out]
                        n240 = call "CVData.vi"("Action"=T3."Write Element", "Array No."=0, "Array Size / Index"=w405, "Data IN"=w412) -> ()  [unwired: 1 in, 2 out]
                        n241 = call "CVData.vi"("Action"=T3."Write Element", "Array No."=u32 1, "Array Size / Index"=w394, "Data IN"=w406) -> ()  [unwired: 1 in, 2 out]
                        n242 = local read "Current reading No."() -> (w409:u32)
                        n243 = Increment(x=w409) -> (x+1=w422:u32)
                        n244 = local write "Current reading No."(w422) -> ()
                      }
                      frame #1 {
                        w455 = u32 5 ("y")
                        # "Update Capacitance/Voltage plots"
                        # "Set minimum in Capacitance (Y) axis in 0 if linear and 1 if logarithmic"
                        # "Update CV plot and show Temperature/Relative Humidity and last 5 readings of Capacitance/Resistance/Voltage"
                        n245 = call "CVData.vi"("Action"=T3."Read Array", "Array No."=1) -> ("Array OUT"=w444:dbl[])  [unwired: 3 in, 1 out]
                        n246 = Array Subset(array=w444, index=0, length=w446) -> (w450:dbl[])
                        n247 = Greater?(x=w446, y=w455) -> (0:w454:bool)
                        n248 = local read "Cscale"() -> (w456:enum16{"1/C^2 [1/nF^2]", "nF", "pF"})
                        n249 = Absolute Value(x=w450) -> (abs(x)=w449:dbl[])
                        n250 = case shown="True" w454 {
                          tunnel: w446 -> [w463 w466]
                          tunnel: w455 -> [_ w465]
                          tunnel: [w463 w465] -> w453
                          tunnel: [0 w464] -> w451
                          frame False {
                          }
                          frame True {
                            n251 = Subtract(x=w466, y=w465) -> (x-y=w464:u32)
                          }
                        }
                        n252 = case shown="..\"1/C^2 [1/nF^2]\"" w456 {
                          tunnel: [w499 w502 w505] -> w461
                          tunnel: w449 -> [w497 w504 w505]
                          frame .."1/C^2 [1/nF^2]" {
                            # "Converts pF to nF^-2"
                            n253 = Array Size(array=w497) -> (size(s)=w498:i32)
                            n254 = for {
                              N: w498 -> [_]
                              tunnel: w497 -> [w501] mode=indexing
                              tunnel: [w500] -> w499 mode=indexing
                              n255 = formula code="y=1000000./(x*x);"("x"=w501) -> ("y"=w500:dbl)
                            }
                          }
                          frame "nF" {
                            # "Converts pF to nF"
                            n256 = Divide(x=w504, y=1000.0) -> (x/y=w502:dbl[])
                          }
                          frame "pF".. {
                          }
                        }
                        n257 = for {
                          N: 5 -> [_]
                          tunnel: w453 -> [w472]
                          tunnel: w451 -> [w471]
                          tunnel: w446 -> [w470]
                          i -> [w468]
                          # "Update \"Last 5 readings:\" CV indicator and T/RH indicators"
                          n258 = call "CVData.vi"("Action"=T3."Read Array", "Array No."=w468) -> ("Array OUT"=w467:dbl[])  [unwired: 3 in, 1 out]
                          n259 = case shown="4.." w468 {
                            tunnel: w472 -> [w475 w479 w484 _ _]
                            tunnel: w471 -> [w476 w480 w485 _ _]
                            tunnel: w467 -> [w474 w478 w486 w490 w495]
                            tunnel: w470 -> [_ _ _ w488 w493]
                            frame ..0 {
                              # "Read Voltage from 1st column"
                              n260 = Array Subset(array=w474, index=w476, length=w475) -> (w473:dbl[])
                              n261 = local write "Volts"(w473) -> ()
                            }
                            frame 1 {
                              # "Read Capacitance from 2nd column"
                              n262 = Array Subset(array=w478, index=w480, length=w479) -> (w477:dbl[])
                              n263 = local write "Capacitance"(w477) -> ()
                            }
                            frame 2 {
                              # "Read Resistance from 3rd column"
                              n264 = Array Subset(array=w486, index=w485, length=w484) -> (w483:dbl[])
                              n265 = Multiply(x=w483, y=0.001) -> (x*y=w482:dbl[])
                              n266 = local write "Resistance"(w482) -> ()
                            }
                            frame 3 {
                              # "Read Temperature from 4th column"
                              n267 = Decrement(x=w488) -> (x-1=w487:u32)
                              n268 = Array Subset(array=w490, index=w487, length=1) -> (w489:dbl[])
                              n269 = local write "Temp."(w489) -> ()
                            }
                            frame 4.. {
                              # "Read Relative Humidity from 5th column"
                              n270 = Decrement(x=w493) -> (x-1=w492:u32)
                              n271 = Array Subset(array=w495, index=w492, length=1) -> (w494:dbl[])
                              n272 = local write "RH"(w494) -> ()
                            }
                          }
                        }
                        n273 = local read "Initial volts [V]"() -> (w459:dbl)
                        n274 = Absolute Value(x=w458) -> (abs(x)=w457:dbl)
                        n275 = property on="Cgraph" class="WFGraph (strict)"() -> ("YScale.Mapping Mode"=w447:u8)  [unwired: 2 in, 2 out]
                        n276 = Bundle("Initial volts [V]"=w459, w457, w461) -> (w448:cluster{"Initial volts [V]":dbl, dbl, dbl[]})  [unwired: 1 in]
                        n277 = local write "Cgraph"(w448) -> ()
                        n278 = property on="Cgraph" class="WFGraph (strict)"("YScale.Minimum"=w447) -> ()  [unwired: 2 in, 2 out]
                      }
                      frame #2 {
                        # "Increase volts and check for end of ramp"
                        # "Increase voltage and check compliance"
                        n279 = local read "Current Volts:"() -> (w512:dbl)
                        n280 = local read "Current Volts:"() -> (w506:dbl)
                        n281 = local read "positive ramp?"() -> (w516:bool)
                        n282 = Quotient & Remainder(x=w512, y=w511) -> (x-y*floor(x/y)=w513:dbl, floor(x/y)=w510:dbl)
                        n283 = Not Equal To 0?(x=w513) -> (x != 0?=w508:bool)
                        n284 = Equal To 0?(x=w510) -> (x = 0?=w509:bool)
                        n285 = case shown="False" w516 {
                          tunnel: w511 -> [w523 w527]
                          tunnel: w520 -> [w524 w530]
                          tunnel: [w522 w529] -> w507
                          tunnel: [w521 w526] -> w519
                          tunnel: w506 -> [w525 w528]
                          frame False {
                            n286 = Subtract(x=w525, y=w524) -> (x-y=w521:dbl)
                            n287 = Greater Or Equal?(x=w521, y=w523) -> (x >= y?=w522:bool)
                          }
                          frame True {
                            n288 = Add(x=w528, y=w530) -> (x+y=w526:dbl)
                            n289 = Less Or Equal?(x=w526, y=w527) -> (x <= y?=w529:bool)
                          }
                        }
                        n290 = Or(x=w508, y=w509) -> ()  [unwired: 1 out]
                        n291 = case shown="True" w507 {
                          tunnel: w519 -> [_ w541]
                          tunnel: [TRUE FALSE] -> w518
                          tunnel: [FALSE w542] -> w517
                          tunnel: w512 -> [_ w539]
                          tunnel: w515 -> [_ w538]
                          tunnel: w514 -> [_ w537]
                          frame False {
                          }
                          frame True {
                            # "Message \"Incrementing volts.\""
                            # "Increase  voltage, check compliance and check IV supply errors"
                            n292 = local read "step [V]"() -> (w535:dbl)
                            n293 = call "SupplyRamp.vi"("error in"=w538, "Requested Voltage"=w541, "Step Size"=w535, "Step Delay"=100, "Supply IN"=w537, "Starting Voltage"=w539) -> ("error out"=w533:errorcluster, "Compliance exceeded"=w542:bool, "Current Voltage"=w536:dbl)  [unwired: 2 in, 1 out]
                            n294 = local write "STATUS 1"("Incrementing volts.") -> ()
                            n295 = property on="Bias On/Off:" class="Bool (strict)"("Blinking"=w542) -> ()  [unwired: 2 in, 2 out]
                            n296 = case shown="No Error" w533 {
                              tunnel: w536 -> [w544 _]
                              frame No Error {
                                n297 = local write "Current Volts:"(w544) -> ()
                              }
                              frame Error {
                              }
                            }
                          }
                        }
                      }
                    }
                  }
                  frame True {
                    w545 = FALSE
                    # "\"ABORT\" button pressed"
                  }
                }
              }
            }
            n298 = case shown="True" w293 {
              frame False {
              }
              frame True {
                n299 = property on="Bias On/Off:" class="Bool (strict)"("Blinking"=TRUE) -> ()  [unwired: 2 in, 2 out]
              }
            }
            n300 = Build Array(w295, w293, "abort", w294) -> (w299:bool[])
            n301 = Or Array Elements(Boolean array=w299) -> (logical OR=w305:bool)
            n302 = Not(x=w305) -> (.not. x?=w304:bool)
          }
        }
        frame True {
          w547 = FALSE
          # "compliance was exceeded when first voltage applied."
          # "Flag compliance as reason for end of run"
          # "Compliance exceeded when first voltage applied"
          n303 = local write "STATUS 1"("Run aborted - compliance exceeded.") -> ()
          n304 = Build Array(w547, TRUE, w547, w547) -> (w548:bool[])
        }
      }
      n305 = Search 1D Array(1D array=w282, element=TRUE) -> (index of element=w280:i32)  [unwired: 1 in]
      n306 = Increment(x=w280) -> (x+1=w279:i32)
      n307 = case shown="1" w279 {
        tunnel: ["" "Run ended normally" "Compliance exceeded" "Run aborted - by user" "Run aborted - Ilimit exceeded"] -> w274
        frame ..0 {
        }
        frame 1 {
        }
        frame 2 {
        }
        frame 3 {
        }
        frame 4.. {
        }
      }
      n308 = Concatenate Strings(w274, "\r\n", "RAMPING DOWN VOLTS") -> (w277:string)
      n309 = global read "QC_RunInformation.vi" "Run info"() -> (w278:T7)
      n310 = Bundle By Name(cluster=w278, "End of Run comment:"=w274) -> (w273:T7)
      n311 = local write "STATUS 1"(w277) -> ()
      n312 = global write "QC_RunInformation.vi" "Run info"(w273) -> ()
    }
    frame #4 {
      # "Ramp down, switch off supply, ask to save data and save jpg of the Front Panel"
      n313 = stacked-sequence {
        frame #0 {
          # "Switch IV supply to STANDBY"
          # "s -> ms"
          # "Ramp down voltage and switch IV supply to standby"
          n314 = global read "QC_MeasurementSetup.vi" "CV Measurement Parameters"() -> (w559:T6)
          n315 = Unbundle By Name(w559) -> ("Supply"=w558:refnum<class "SupplyControl.lvclass">, "Ramp down Interval [s]"=w552:i32, "Ramp down steps [V]"=w551:dbl, "Switching"=w554:refnum<class "Switching.lvclass">, "Matrix used?"=w553:bool)
          n316 = local read "Current Volts:"() -> (w564:dbl)
          n317 = Multiply(x=w552, y=1000) -> (x*y=w561:i32)
          n318 = call "SupplyRamp.vi"("Requested Voltage"=0.0, "Step Size"=w551, "Step Delay"=w561, "Supply IN"=w558, "Starting Voltage"=w564) -> ("error out"=w556:errorcluster, "Supply OUT"=w557:refnum<class "SupplyControl.lvclass">, "Current Voltage"=w562:dbl)  [unwired: 3 in, 1 out]
          n319 = local write "Current Volts:"(w562) -> ()
          n320 = call-dynamic "Supply_Stby.vi"("error in (no error)"=w556, "SupplyControl in"=w557) -> ("error out"=w555:errorcluster)  [unwired: 8 in, 1 out]
          n321 = case shown="True" w553 {
            tunnel: w554 -> [_ w569]
            tunnel: w555 -> [_ w568]
            frame False {
            }
            frame True {
              # "CLOSE Switching Matrix"
              # "RESET Switching  Matrix"
              n322 = call-dynamic "MatrixSwitch.vi"("error in (no error)"=w568, "Action"=T4."Reset", "Switching in"=w569) -> ("error out"=w565:errorcluster, "Switching out"=w566:refnum<class "Switching.lvclass">)  [unwired: 6 in, 1 out]
              n323 = call-dynamic "Close.vi"("error in (no error)"=w565, "Switching in"=w566) -> ()  [unwired: 8 in, 2 out]
            }
          }
        }
        frame #1 {
          w574 = 0
          # "\"QUIT\" and \"Save & QUIT\" buttons \nenabled (Disabled=0)"
          # "\"Current Volts\" indicator back to 0.00 V"
          # "\"ABORT\" button disanabled \nand dimmed (Disabled=2)"
          # "\"Bias  On/Off\" indicator in Off (red)"
          # "Reset \"Current Volts\" and \"Bias On/Off\" indicators, \"ABORT\" button disabled and \"QUIT\"/\"Save & QUIT\" buttons enabled"
          n324 = property on="Quit & Save" class="Bool"("DisabledEnum"=w574) -> ()  [unwired: 2 in, 2 out]
          n325 = property on="quit (no save)" class="Bool"("DisabledEnum"=w574) -> ()  [unwired: 2 in, 2 out]
          n326 = local write "Current Volts:"(0.0 ("Current Volts:")) -> ()
          n327 = property on="abort" class="Bool (strict)"("DisabledEnum"=2) -> ()  [unwired: 2 in, 2 out]
          n328 = local write "Bias On/Off:"(FALSE ("Visible")) -> ()
          n329 = local write "STATUS 1"("Run finished. \nSave data?" ("STATUS 1")) -> ()
        }
        frame #2 {
          # "Save  jpg  image of the Front Panel"
          n330 = Current VI's Path() -> (path=w576:path)
          n331 = call "SaveJPEG.vi"("Test"="CV", "File Path Control"=w576) -> ()  [unwired: 1 in, 2 out]
        }
      }
    }
    frame #5 {
      # "*WARNING*: \"Done!\" indicator in \nFront Panel hidden."
      # "Switch off Arduino if used for T/RH measurement"
      # "Display and save data"
      n332 = global read "QC_MeasurementSetup.vi" "CV Measurement Parameters"() -> (w585:T6)
      n333 = local read "Scales"() -> (w587:T1)
      n334 = local read "Cscale"() -> (w586:enum16{"1/C^2 [1/nF^2]", "nF", "pF"})
      n335 = while {
        shift-left: w586 -> [w634]
        shift-right: [w633] -> _
        shift-left: w587 -> [w636]
        shift-right: [w635] -> _
        tunnel: ["Quit & Save"] -> w589
        tunnel: ["quit (no save)"] -> w588
        stop <- w631 continue-if-true
        # "Loop and await decision on whether to save or junk data"
        n336 = local read "Scales"() -> (w635:T1)
        n337 = local read "Cscale"() -> (w633:enum16{"1/C^2 [1/nF^2]", "nF", "pF"})
        n338 = Not Equal?(x=w636, y=w635) -> (x != y?=w629:bool)
        n339 = Not Equal?(x=w634, y=w633) -> (x != y?=w628:bool)
        n340 = case shown="True" w629 {
          tunnel: w635 -> [_ w663]
          frame False {
          }
          frame True {
            # "Allow to change the CV plot representation (Linear=0, Logarithmic=1)"
            n341 = case shown="\"Log - Lin\"" w663 {
              tunnel: [w664 1 0 w669] -> w662
              tunnel: [w664 0 1 w669] -> w661
              frame .."Lin - Lin" {
                w664 = 0
              }
              frame "Log - Lin" {
              }
              frame "Lin - Log" {
              }
              frame "Log - log".. {
                w669 = 1
              }
            }
            n342 = property on="Cgraph" class="WFGraph (strict)"("X Scale.Mapping Mode"=w662) -> ()  [unwired: 2 in, 2 out]
            n343 = property on="Cgraph" class="WFGraph (strict)"("Y Scale.Mapping Mode"=w661, "YScale.Minimum"=w661) -> ()  [unwired: 2 in, 2 out]
          }
        }
        n344 = case shown="True" w628 {
          tunnel: w633 -> [_ w641]
          frame False {
          }
          frame True {
            # "Set minimum in Current (Y) axis in 0 if linear and 1 if logarithmic"
            # "Allow to change the Capacitance scale (pF, nF^-2 or nF)"
            n345 = global read "QC_MeasurementSetup.vi" "CV Measurement Parameters"() -> (w643:T6)
            n346 = property on="Cgraph" class="WFGraph (strict)"() -> ("YScale.Mapping Mode"=w644:u8)  [unwired: 2 in, 2 out]
            n347 = property on="Cgraph" class="WFGraph (strict)"("YScale.Minimum"=w644) -> ()  [unwired: 2 in, 2 out]
            n348 = Unbundle By Name(w643) -> ("Initial Voltage [V]"=w646:dbl, "Step Size [V]"=w648:dbl, "Number Of Steps"=w645:u32)
            n349 = Absolute Value(x=w648) -> (abs(x)=w647:dbl)
            n350 = call "CVData.vi"("Action"=T3."Read Array", "Array No."=u32 1 ("Action")) -> ("Array OUT"=w637:dbl[])  [unwired: 3 in, 1 out]
            n351 = Array Subset(array=w637, index=0, length=w645) -> (w649:dbl[])
            n352 = Absolute Value(x=w649) -> (abs(x)=w642:dbl[])
            n353 = case shown="..\"1/C^2 [1/nF^2]\"" w641 {
              tunnel: [w654 w657 w660] -> w640
              tunnel: w642 -> [w652 w659 w660]
              frame .."1/C^2 [1/nF^2]" {
                n354 = Array Size(array=w652) -> (size(s)=w653:i32)
                n355 = for {
                  N: w653 -> [_]
                  tunnel: w652 -> [w656] mode=indexing
                  tunnel: [w655] -> w654 mode=indexing
                  n356 = formula code="y=1000000./(x*x);"("x"=w656) -> ("y"=w655:dbl)
                }
              }
              frame "nF" {
                n357 = Divide(x=w659, y=1000.0) -> (x/y=w657:dbl[])
              }
              frame "pF".. {
              }
            }
            n358 = Bundle("Initial Voltage [V]"=w646, w647, w640) -> (w650:cluster{"Initial Voltage [V]":dbl, dbl, dbl[]})  [unwired: 1 in]
            n359 = local write "Cgraph"(w650) -> ()
          }
        }
        n360 = Not Or(1:"quit (no save)", 2:"Quit & Save") -> (0:w631:bool)
      }
      n361 = Unbundle By Name(w585) -> ("Temperature Readout"=w584:enum16{"Read Arduino", "Enter manually"}, "Arduino"=w578:refnum<class "ArduinoControl.lvclass">)
      n362 = case shown="\"Read Arduino\"" w584 {
        tunnel: w578 -> [_ w627]
        frame "Enter manually", Default {
        }
        frame "Read Arduino" {
          n363 = call "ArduinoClose.vi"("ArduinoControl in"=w627) -> ()  [unwired: 9 in, 2 out]
        }
      }
      n364 = case shown="True" w588 {
        tunnel: [FALSE w671] -> w590
        frame False {
        }
        frame True {
          n365 = Two Button Dialog(message="Are you sure you don't want to save the data?", 1:"Quit" ("F button name (\"Cancel\")"), 2:"Save data" ("T button name (\"OK\")")) -> (T button?=w671:bool)
        }
      }
      n366 = Or(x=w589, y=w590) -> (x .or. y?=w583:bool)
      n367 = flat-sequence {
        tunnel: w583 -> [w592]
        tunnel: [w592] -> w579
        tunnel: [TRUE] -> w577
        frame #0 {
          # "Extract Full Depletion Voltage"
          n368 = global read "QC_MeasurementSetup.vi" "CV Measurement Parameters"() -> (w602:T6)
          n369 = Unbundle By Name(w602) -> ("V_depletion Limit [V]"=w594:dbl, "Number Of Steps"=w597:u32)
          n370 = call "ScanFeedback.vi"("measurement type"=T5."CV") -> ("V depletion"=w596:dbl)  [unwired: 4 in, 4 out]
          n371 = Absolute Value(x=w596) -> (abs(x)=w595:dbl)
          n372 = Absolute Value(x=w594) -> (abs(x)=w593:dbl)
          n373 = Less Or Equal?(x=w595, y=w593) -> (x <= y?=w598:bool)
          n374 = case shown="True" w592 {
            tunnel: ["" w626] -> w603
            tunnel: [_ w611] -> w601
            tunnel: w597 -> [_ _]
            frame False {
            }
            frame True {
              w609 = T3."Read Array" ("Action")
              # "Show \"Saving Data ...\" message"
              # "Save data in file"
              n375 = local write "STATUS 1"("Saving Data ...") -> ()
              n376 = call "CVData.vi"("Action"=w609, "Array No."=u32 0 ("Action")) -> ("Array OUT"=w617:dbl[])  [unwired: 3 in, 1 out]
              n377 = call "CVData.vi"("Action"=w609, "Array No."=u32 1 ("Action")) -> ("Array OUT"=w616:dbl[])  [unwired: 3 in, 1 out]
              n378 = call "CVData.vi"("Action"=w609, "Array No."=u32 2 ("Action")) -> ("Array OUT"=w607:dbl[])  [unwired: 3 in, 1 out]
              n379 = Multiply(x=w607, y=0.001) -> (x*y=w606:dbl[])
              n380 = Build Array(w617, w616, w606) -> (w615:dbl[][])
              n381 = call "CVData.vi"("Action"=w609, "Array No."=u32 4 ("Action")) -> ("Array OUT"=w623:dbl[])  [unwired: 3 in, 1 out]
              n382 = call "CVData.vi"("Action"=w609, "Array No."=u32 3 ("Action")) -> ("Array OUT"=w622:dbl[])  [unwired: 3 in, 1 out]
              n383 = Transpose 2D Array(2D array=w615) -> (transposed array=w614:dbl[][])
              n384 = call <vilib>:"Std Deviation and Variance.vi"("X"=w623) -> ("mean"=w612:dbl)  [unwired: 1 in, 2 out]
              n385 = call <vilib>:"Std Deviation and Variance.vi"("X"=w622) -> ("mean"=w613:dbl)  [unwired: 1 in, 2 out]
              n386 = call "SaveDataFile.vi"("Data Array"=w614, "Temperature"=w613, "Humidity"=w612, "Array Titles"="Voltage[V] Capacitance[pF] Resistance[kOhm]", "Strip Segment"="") -> ("Path + Filename OUT"=w626:string, "Error Out"=w611:errorcluster)  [unwired: 7 in, 2 out]
            }
          }
          n387 = call "WriteLogFile.vi"("Automatic warning"="", "Data File"=w603, "Error In"=w601, "DUT passed?"=w598, "Value TechSpec criteria"=w596, "Files saved?"=w592) -> ()  [unwired: 5 in, 1 out]
        }
      }
      n388 = Select(t="Run finished.\nData saved." ("STATUS 1"), s=w579, f="Run finished.\nData not saved." ("STATUS 1")) -> (s? t:f=w582:string)
      n389 = local write "STATUS 1"(w582) -> ()
      "Done!" <- w577
    }
  }
